vi "Launch SessionCore (Client).vi"(8 "error in (no error)":errorcluster, 11 "Session in":refnum<class "Session.lvclass">) -> (0 "error out":errorcluster, 2 "Session ID":i32, 3 "Session out":refnum<class "Session.lvclass">)   [LabVIEW 2013]
uses:
  Session.lvclass
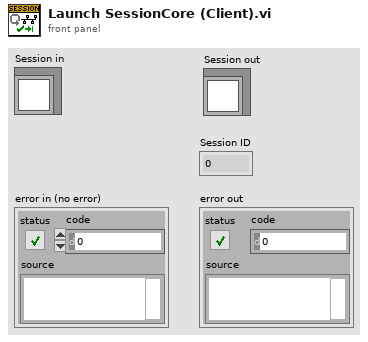
[diagram p1: front panel]
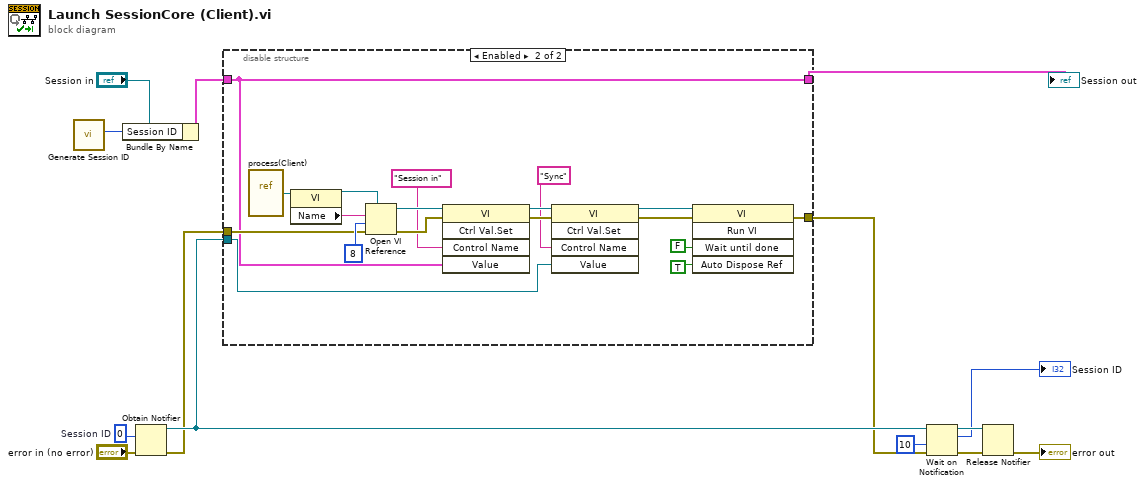
[diagram p0: block diagram]
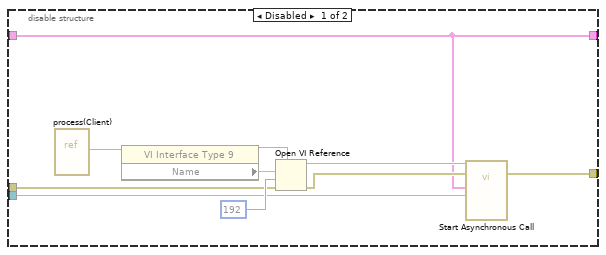
[diagram p2: hidden frame]
diagram:
  w9 = 0  # Session ID
  n1 = call "Generate Session ID.vi"() -> ("Session ID"=w3:i32)  [unwired: 11 in]
  n2 = Bundle By Name(cluster="Session in", "Session ID"=w3) -> (w1:cluster{})
  n3 = Obtain Notifier(notification data type=w9, error in (no error)="error in (no error)") -> (notifier out=w6:refnum<notifier>, error out=w5:errorcluster)  [unwired: 2 in, 1 out]
  n4 = disable-structure shown="Enabled" {
    disable-tunnel: w5 -> [w19 w39]
    disable-tunnel: w1 -> [w17 w32]
    disable-tunnel: [w18 w36] -> w4
    disable-tunnel: [w17 w32] -> w7
    disable-tunnel: w6 -> [w15 w27]
    frame Disabled {
      n5 = vi-ref "process(Client).vi"() -> (w16:refnum<vi>)
      n6 = property class="VI Interface Type 9"(reference=w16) -> (reference out=w23:refnum<vi>, "Name"=w24:string)  [unwired: 1 in, 1 out]
      n7 = Open VI Reference(type specifier VI Refnum (for type only)=w23, vi path=w24, options=192, error in (no error)=w19) -> (vi reference=w22:refnum<vi>, error out=w21:errorcluster)  [unwired: 2 in]
      n8 = call-by-ref "Start Asynchronous Call"(reference=w22, error in=w21, "Sync"=w15, "Session in"=w17) -> (error out=w18:errorcluster)  [unwired: 8 in, 3 out]
    }
    frame Enabled {
      n9 = vi-ref "process(Client).vi"() -> (w31:refnum<vi>)
      n10 = property class="VI"(reference=w31) -> (reference out=w41:refnum<vi>, "Name"=w42:string)  [unwired: 1 in, 1 out]
      n11 = Open VI Reference(type specifier VI Refnum (for type only)=w41, vi path=w42, options=8, error in (no error)=w39) -> (vi reference=w34:refnum<vi>, error out=w35:errorcluster)  [unwired: 2 in]
      n12 = invoke class="VI" method="Ctrl Val.Set"(reference=w34, error in=w35, "Control Name"="Session in", "Value"=w32) -> (reference out=w30:refnum<vi>, error out=w29:errorcluster)  [unwired: 1 in, 3 out]
      n13 = invoke class="VI" method="Ctrl Val.Set"(reference=w30, error in=w29, "Control Name"="Sync", "Value"=w27) -> (reference out=w26:refnum<vi>, error out=w25:errorcluster)  [unwired: 1 in, 3 out]
      n14 = invoke class="VI" method="Run VI"(reference=w26, error in=w25, "Wait until done"=FALSE ("Wait Until Done"), "Auto Dispose Ref"=TRUE ("Auto Dispose Reference")) -> (error out=w36:errorcluster)  [unwired: 1 in, 4 out]
    }
  }
  "Session out" <- w7
  n15 = Wait on Notification(notifier=w6, timeout in ms (-1)=10, error in (no error)=w4) -> (notifier out=w10:refnum<notifier>, notification=→"Session ID":i32, error out=w12:errorcluster)  [unwired: 1 in, 1 out]
  n16 = Release Notifier(notifier=w10, error in (no error)=w12) -> (error out=→"error out":errorcluster)  [unwired: 1 in, 2 out]
